vi "setILCData.vi"(10 "ILCData":T1 {"Responses"."ReadCalibration" items=["OK", "IllegalFunction", "IllegalDataAddress", "IllegalDataValue", "SlaveDeviceFailure", "Acknowledge", "SlaveDeviceBusy", "NegativeAcknowledge", "MemoryParityError", "GatewayPathUnavailable", "GatewayTargetDeviceFailedToRespond"]; "Responses"."ReadDAC" items=["OK", "IllegalFunction", "IllegalDataAddress", "IllegalDataValue", "SlaveDeviceFailure", "Acknowledge", "SlaveDeviceBusy", "NegativeAcknowledge", "MemoryParityError", "GatewayPathUnavailable", "GatewayTargetDeviceFailedToRespond"]; "Responses"."ADCOffsetSensitivity" items=["OK", "IllegalFunction", "IllegalDataAddress", "IllegalDataValue", "SlaveDeviceFailure", "Acknowledge", "SlaveDeviceBusy", "NegativeAcknowledge", "MemoryParityError", "GatewayPathUnavailable", "GatewayTargetDeviceFailedToRespond"]; "Responses"."ADCScanRate" items=["OK", "IllegalFunction", "IllegalDataAddress", "IllegalDataValue", "SlaveDeviceFailure", "Acknowledge", "SlaveDeviceBusy", "NegativeAcknowledge", "MemoryParityError", "GatewayPathUnavailable", "GatewayTargetDeviceFailedToRespond"]; "Responses"."Reset" items=["OK", "IllegalFunction", "IllegalDataAddress", "IllegalDataValue", "SlaveDeviceFailure", "Acknowledge", "SlaveDeviceBusy", "NegativeAcknowledge", "MemoryParityError", "GatewayPathUnavailable", "GatewayTargetDeviceFailedToRespond"]; "Responses"."SetTemporaryAddress" items=["OK", "IllegalFunction", "IllegalDataAddress", "IllegalDataValue", "SlaveDeviceFailure", "Acknowledge", "SlaveDeviceBusy", "NegativeAcknowledge", "MemoryParityError", "GatewayPathUnavailable", "GatewayTargetDeviceFailedToRespond"]; "Responses"."ILCMode" items=["OK", "IllegalFunction", "IllegalDataAddress", "IllegalDataValue", "SlaveDeviceFailure", "Acknowledge", "SlaveDeviceBusy", "NegativeAcknowledge", "MemoryParityError", "GatewayPathUnavailable", "GatewayTargetDeviceFailedToRespond"]; "Responses"."ReportServerStatus" items=["OK", "IllegalFunction", "IllegalDataAddress", "IllegalDataValue", "SlaveDeviceFailure", "Acknowledge", "SlaveDeviceBusy", "NegativeAcknowledge", "MemoryParityError", "GatewayPathUnavailable", "GatewayTargetDeviceFailedToRespond"]; "Responses"."ReportServerID" items=["OK", "IllegalFunction", "IllegalDataAddress", "IllegalDataValue", "SlaveDeviceFailure", "Acknowledge", "SlaveDeviceBusy", "NegativeAcknowledge", "MemoryParityError", "GatewayPathUnavailable", "GatewayTargetDeviceFailedToRespond"]; "Telemetry"."ADCScanRate" items=["50 Hz"=0, "60 Hz"=1, "100 Hz"=2, "120 Hz"=3, "200 Hz"=4, "240 Hz"=5, "300 Hz"=6, "400 Hz"=7, "480 Hz"=8, "600 Hz"=9, "1200 Hz"=10, "2400 Hz"=11, "4800 Hz"=12, "No Change"=255]; "Command"."ADCScanRate" items=["50 Hz"=0, "60 Hz"=1, "100 Hz"=2, "120 Hz"=3, "200 Hz"=4, "240 Hz"=5, "300 Hz"=6, "400 Hz"=7, "480 Hz"=8, "600 Hz"=9, "1200 Hz"=10, "2400 Hz"=11, "4800 Hz"=12, "No Change"=255]}, 11 "ILC in":refnum<class "ILC.lvclass">) -> (3 "ILC out":refnum<class "ILC.lvclass">)   [LabVIEW 2015, in "RTILC.lvlib" / "ILC.lvclass"]
uses:
  ILC.lvclass
  DataTypes/ILCData.ctl
  DataTypes/ILCConstants.ctl
  DataTypes/ILCCommand.ctl
  DataTypes/ILCScanRates.ctl
  DataTypes/ILCTelemetry.ctl
  DataTypes/ILCResponses.ctl
  Common_RT_Modbus/DataTypes/ExceptionCodes.ctl
  ILC.lvclass/ILC.ctl
  RTILC.lvlib
  Common_RT_Modbus/RTModbus.lvlib
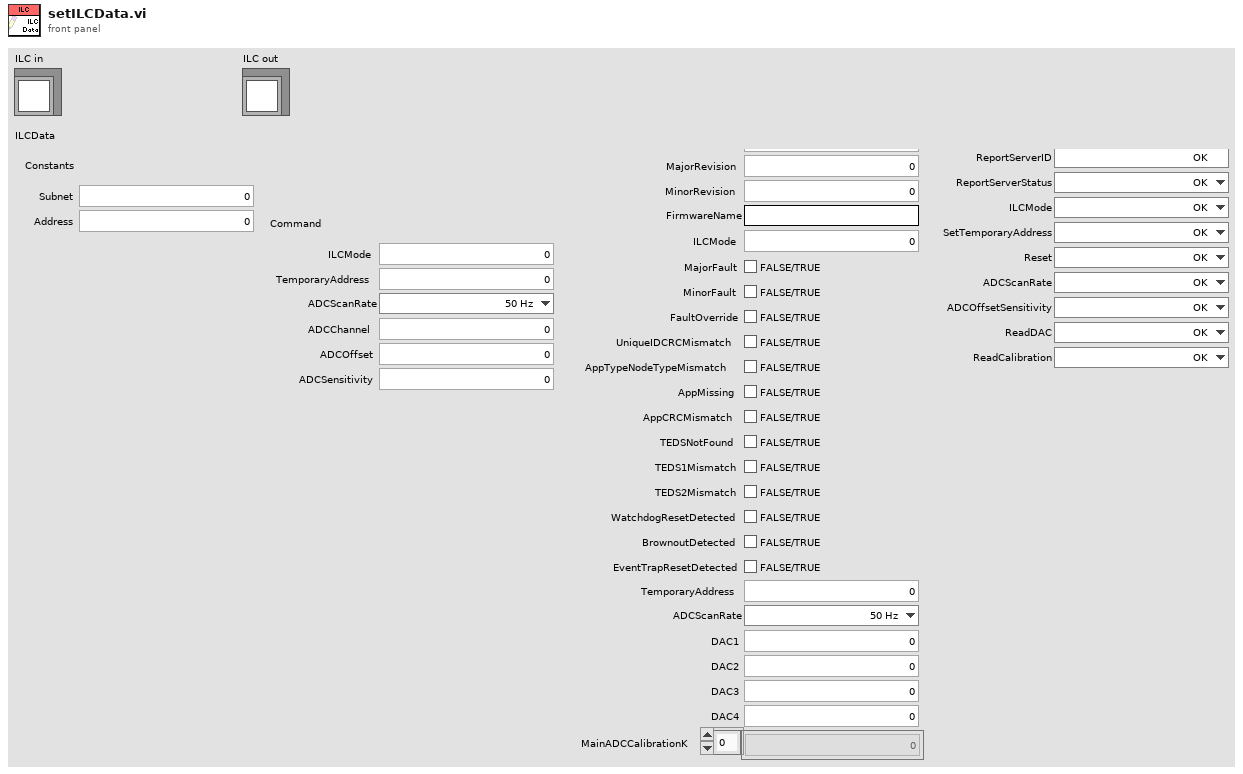
[diagram p1: front panel]
types:
  T1 = typedef "RTILC.lvlib/ILCData.ctl" = cluster{"Constants":T2, "Command":T3, "Telemetry":T5, "Responses":T6}
  T2 = typedef "RTILC.lvlib/ILCConstants.ctl" = cluster{"Subnet":u8, "Address":u8}
  T3 = typedef "RTILC.lvlib/ILCCommand.ctl" = cluster{"ILCMode":u16, "TemporaryAddress":u8, "ADCScanRate":T4, "ADCChannel":u8, "ADCOffset":sgl, "ADCSensitivity":sgl}
  T4 = typedef "RTILC.lvlib/ILCScanRates.ctl" = u8
  T5 = typedef "RTILC.lvlib/ILCTelemetry.ctl" = cluster{"UniqueID":u64, "FirmwareType":u8, "NetworkNodeType":u8, "ILCOption":u8, "NetworkNodeOption":u8, "MajorRevision":u8, "MinorRevision":u8, "FirmwareName":string, "ILCMode":u16, "MajorFault":bool, "MinorFault":bool, "FaultOverride":bool, "UniqueIDCRCMismatch":bool, "AppTypeNodeTypeMismatch":bool, "AppMissing":bool, "AppCRCMismatch":bool, "TEDSNotFound":bool, "TEDS1Mismatch":bool, "TEDS2Mismatch":bool, "WatchdogResetDetected":bool, "BrownoutDetected":bool, "EventTrapResetDetected":bool, "TemporaryAddress":u8, "ADCScanRate":T4, "DAC1":u16, "DAC2":u16, "DAC3":u16, "DAC4":u16, "MainADCCalibrationK":sgl[], "MainSensorOffset":sgl[], "MainSensorSensitivity":sgl[], "BackupADCCalibrationK":sgl[], "BackupSensorOffset":sgl[], "BackupSensorSensitivity":sgl[]}
  T6 = typedef "RTILC.lvlib/ILCResponses.ctl" = cluster{"ReportServerID":T7, "ReportServerStatus":T7, "ILCMode":T7, "SetTemporaryAddress":T7, "Reset":T7, "ADCScanRate":T7, "ADCOffsetSensitivity":T7, "ReadDAC":T7, "ReadCalibration":T7}
  T7 = typedef "RTModbus.lvlib/ExceptionCodes.ctl" = u16
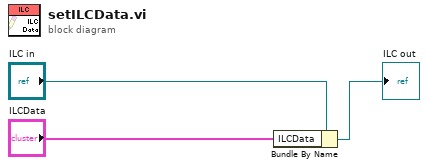
[diagram p0: block diagram]
diagram:
  n1 = Bundle By Name(cluster="ILC in", "ILCData"="ILCData") -> (→"ILC out":refnum<class "ILC.lvclass">)
